vi "Win32Test.vi"() -> ()   [LabVIEW 2016]
uses:
  CAN_Info.ctl
  CAN_BaudInfo.ctl
  CAN_FrameInfo.ctl
  BusStatistics/TLIBCANBusStatistics_Ctrl.ctl
  MessageInfo.ctl
panel:
  out "tsapp_delete_cyclic_msg_can":i32
  in  "AAppChannel":i32(ring) items=["CHN1", "CHN2", "CHN3", "CHN4", "CHN5", "CHN6", "CHN7", "CHN8", "CHN9", "CHN10", "CHN11", "CHN12", "CHN13", "CHN14", "CHN15", "CHN16", "CHN17", "CHN18", "CHN19", "CHN20", "CHN21", "CHN22", "CHN23", "CHN24", "CHN25", "CHN26", "CHN27", "CHN28", "CHN29", "CHN30", "CHN31", "CHN32"]
  in  "删除周期消息":bool
  in  "周期消息":T1 {"ADLC" max=64; "AID" max=536870911}
  in  "添加周期发送消息":bool
  out "tsapp_add_cyclic_msg_can":i32
  in  "消息周期":sgl=10.0
  out "接收的数据":T2[](array[typedef])
  in  "空白按钮":bool
  in  "查询内容":u16(ring) items=["获取网络名称"=0, "获取dbc文件名"=1, "获取协议类型，0=CAN、1=J1939"=2, "获取信号表数量"=10, "获取CAN报文表数量"=11, "获取CANFD报文表数量"=12, "获取CANJ1939报文表数量"=13, "获取节点表数量"=14, "获取环境变量表数量"=15, "获取取值表数量"=16, "获取信号表中第idx信号所在的报文标识符"=20, "获取信号表中第idx信号值类型"=21, "获取信号表中第idx信号是否是Motorola"=22, "获取信号表中第idx信号所带的取值表在取值表列表中的索引"=23, "获取信号表中第idx信号Mux类型"=24, "获取信号表中第idx信号作为multiplexor的值"=25, "获取信号表中第idx信号在报文中的起始位"=26, "获取信号表中第idx信号的信号长度"=27, "获取信号表中第idx信号放大因子"=28, "获取信号表中第idx信号偏移量"=29, "获取信号表中第idx信号初始值"=30, "获取信号表中第idx信号最小值"=31, "获取信号表中第idx信号最大值"=32, "获取信号表中第idx信号名称"=33, "获取信号表中第idx信号单位"=34, "获取信号表中第idx信号注释"=35, "获取信号表中第idx信号所在的报文在报文表中的索引"=36, "获取信号表中第idx信号所在的报文的类型"=37, "获取信号表中第idx信号全部属性"=38, "获取CAN报文表中第idx报文类型"=40, "获取CAN报文表中第idx报文数据长度"=41, "获取CAN报文表中第idx报文标识符"=42, "获取CAN报文表中第idx报文周期"=43, "获取CAN报文表中第idx报文名称"=44, "获取CAN报文表中第idx报文注释"=45, "获取CAN报文表中第idx报文对应的发送节点的索引"=46, "获取CAN报文表中第idx报文拥有的信号数量"=47, "获取CAN报文表中第idx报文中第subidx信号在信号表中的索引"=48, "获取CAN报文表中第idx报文全部属性"=49, "获取CANFD报文表中第idx报文属性"=60, "获取CANFD报文表中第idx报文数据长度"=61, "获取CANFD报文表中第idx报文标识符"=62, "获取CANFD报文表中第idx报文周期"=63, "获取CANFD报文表中第idx报文名称"=64, "获取CANFD报文表中第idx报文注释"=65, "获取CANFD报文表中第idx报文对应的发送节点的索引"=66, "获取CANFD报文表中第idx报文拥有的信号数量"=67, "获取CANFD报文表中第idx报文中第subidx信号在信号表中的索引"=68, "获取CANFD报文表中第idx报文BRS"=69, "获取CANFD报文表中第idx报文全部属性"=70, "获取J1939报文表中第idx报文类型"=80, "获取J1939报文表中第idx报文数据长度"=81, "获取J1939报文表中第idx报文标识符"=82, "获取J1939报文表中第idx报文周期"=83, "获取J1939报文表中第idx报文名称"=84, "获取J1939报文表中第idx报文注释"=85, "获取J1939报文表中第idx报文对应的发送节点的索引"=86, "获取J1939报文表中第idx报文拥有的信号数量"=87, "获取J1939报文表中第idx报文中第subidx信号在信号表中的索引"=88, "获取CAN报文表中第idx报文全部属性"=89, "获取节点表中第idx节点地址"=100, "获取节点表中第idx节点名称"=101, "获取取值表中第idx取值表所包含的值数量"=140, "获取取值表中第idx取值表名称"=141, "获取取值表中第idx取值表中第subidx的值"=142, "获取取值表中第idx取值表全部属性"=143]
  in  "查询dbc":bool
  in  "清除总线统计":bool
  out "TLIBCANBusStatistics_Ctrl":T3
  in  "开启blf记录":bool
  in  "Blf文件路径":path=path "D:/LabviewWorkSpace/海卓项目资料/SFCV FCURig 文件夹/BottomLevel/TS_CANDrive/Test_blf/UserBlf.blf"
  in  "使能统计功能":bool
  out "out AId":u32
  in  "ASupportedChannelsBased0":string
  in  "路径":path
  in  "加载dbc":bool
  in  "错误输入":errorcluster caption="错误输出"
  out "错误输出":errorcluster
  out "ConnectSeccessfully":bool
  in  "初始化CAN通道":bool
  out "接收总数":i32
  in  "发送通道":i32(ring) items=["CHN1", "CHN2", "CHN3", "CHN4", "CHN5", "CHN6", "CHN7", "CHN8", "CHN9", "CHN10", "CHN11", "CHN12", "CHN13", "CHN14", "CHN15", "CHN16", "CHN17", "CHN18", "CHN19", "CHN20", "CHN21", "CHN22", "CHN23", "CHN24", "CHN25", "CHN26", "CHN27", "CHN28", "CHN29", "CHN30", "CHN31", "CHN32"]
  in  "发送数据帧信息":T1={"AID"=1234, "AIsExt"=enum."STD", "AIsRemote"=enum."Data", "ADLC"=5, "ADataArray"=[0, 0, 10, 96, 8, 8]} {"ADLC" max=64; "AID" max=536870911}
  in  "配置波特率":T4={"ABaudrateKbps"=500.0, "AListenOnly"=enum."Normal", "Int120Ohm"=enum."Enable", "EnableChannel"=enum."Enable", "AAppChannel"=0, "硬件类型"=8, "AHwChannel"=0} {"AHwChannel" items=["CHN1", "CHN2", "CHN3", "CHN4", "CHN5", "CHN6", "CHN7", "CHN8", "CHN9", "CHN10", "CHN11", "CHN12", "CHN13", "CHN14", "CHN15", "CHN16", "CHN17", "CHN18", "CHN19", "CHN20", "CHN21", "CHN22", "CHN23", "CHN24", "CHN25", "CHN26", "CHN27", "CHN28", "CHN29", "CHN30", "CHN31", "CHN32"]; "硬件类型" items=["BUS_UNKNOWN_TYPE", "TS_TCP_DEVICE", "XL_USB_DEVICE", "TS_USB_DEVICE", "PEAK_USB_DEVICE", "KVASER_USB_DEVICE", "ZLG_USB_DEVICE", "ICS_USB_DEVICE", "TS_TC1005_DEVICE"]; "AAppChannel" items=["CHN1", "CHN2", "CHN3", "CHN4", "CHN5", "CHN6", "CHN7", "CHN8", "CHN9", "CHN10", "CHN11", "CHN12", "CHN13", "CHN14", "CHN15", "CHN16", "CHN17", "CHN18", "CHN19", "CHN20", "CHN21", "CHN22", "CHN23", "CHN24", "CHN25", "CHN26", "CHN27", "CHN28", "CHN29", "CHN30", "CHN31", "CHN32"]}
  in  "CAN_CardProperties":T5={"应用程序名"="APP", "CAN使用通道数"=5, "LIN使用通道数"=0} {"LIN使用通道数" max=5; "CAN使用通道数" max=5}
  in  "停止":bool
  # "win32目前没有dbc属性获取，\n需要.net方式"
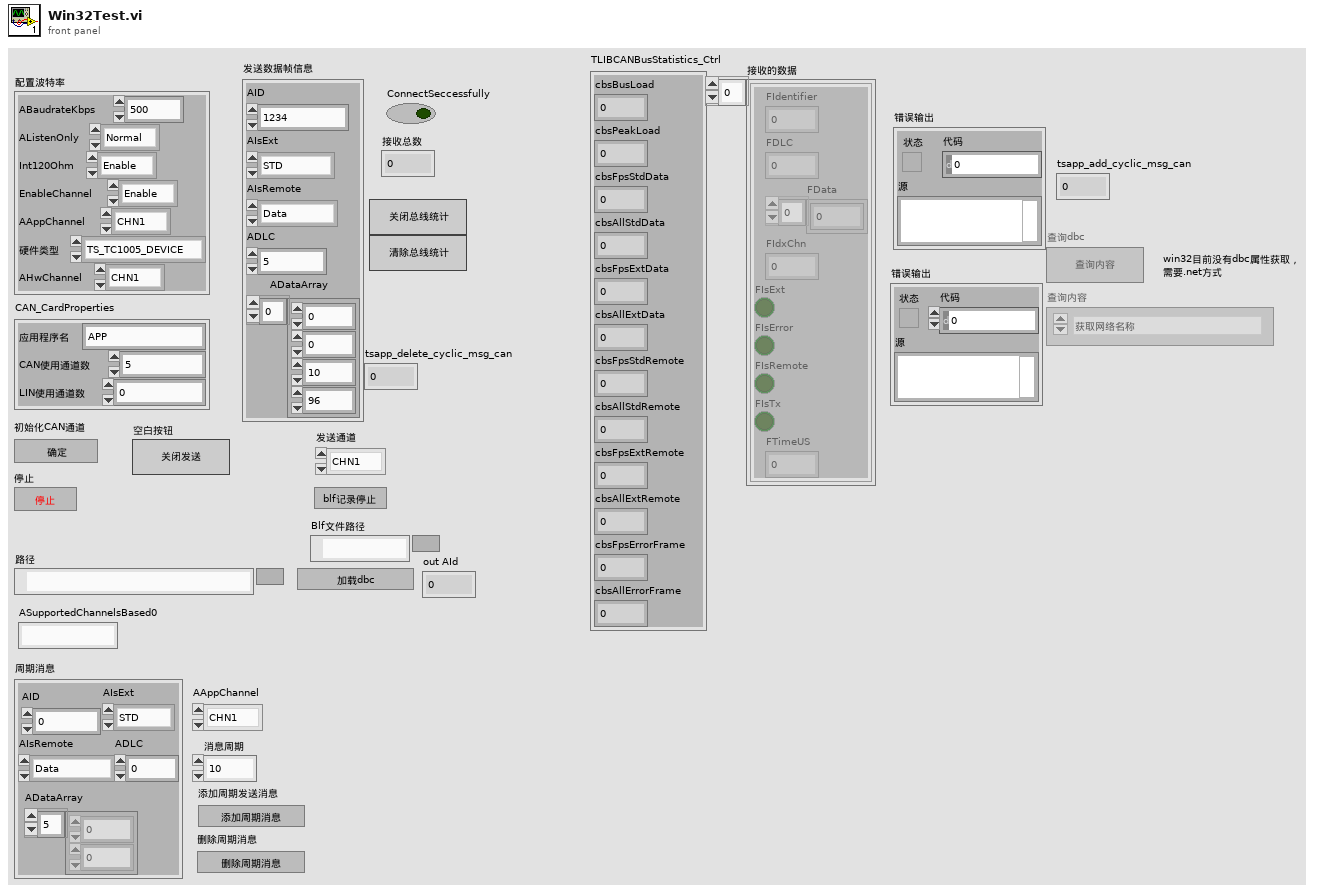
[diagram p1: front panel]
types:
  T1 = typedef "CAN_FrameInfo.ctl" = cluster{"AID":u32, "AIsExt":enum16{"STD", "EXT"}, "AIsRemote":enum16{"Data", "Remote"}, "ADLC":u8, "ADataArray":u8[]}
  T2 = typedef "MessageInfo.ctl" = cluster{"FIdentifier":i32, "FDLC":u8, "FData":u8[], "FIdxChn":u8, "FIsExt":bool, "FIsError":bool, "FIsRemote":bool, "FIsTx":bool, "FTimeUS":u64}
  T3 = typedef "TLIBCANBusStatistics_Ctrl.ctl" = cluster{"cbsBusLoad":dbl, "cbsPeakLoad":dbl, "cbsFpsStdData":dbl, "cbsAllStdData":dbl, "cbsFpsExtData":dbl, "cbsAllExtData":dbl, "cbsFpsStdRemote":dbl, "cbsAllStdRemote":dbl, "cbsFpsExtRemote":dbl, "cbsAllExtRemote":dbl, "cbsFpsErrorFrame":dbl, "cbsAllErrorFrame":dbl}
  T4 = typedef "CAN_BaudInfo.ctl" = cluster{"ABaudrateKbps":sgl, "AListenOnly":enum16{"Normal", "ListenOnly"}, "Int120Ohm":enum16{"Disable", "Enable"}, "EnableChannel":enum16{"Disable", "Enable"}, "AAppChannel":i32, "硬件类型":i32, "AHwChannel":i32}
  T5 = typedef "CAN_Info.ctl" = cluster{"应用程序名":string, "CAN使用通道数":u8, "LIN使用通道数":u8}
  T6 = enum16{"CHAN1", "CHAN2", "CHAN3", "CHAN4", "CHAN5", "CHAN6", "CHAN7", "CHAN8", "CHAN9", "CHAN10", "CHAN11", "CHAN12", "CHAN13", "CHAN14", "CHAN15", "CHAN16"}
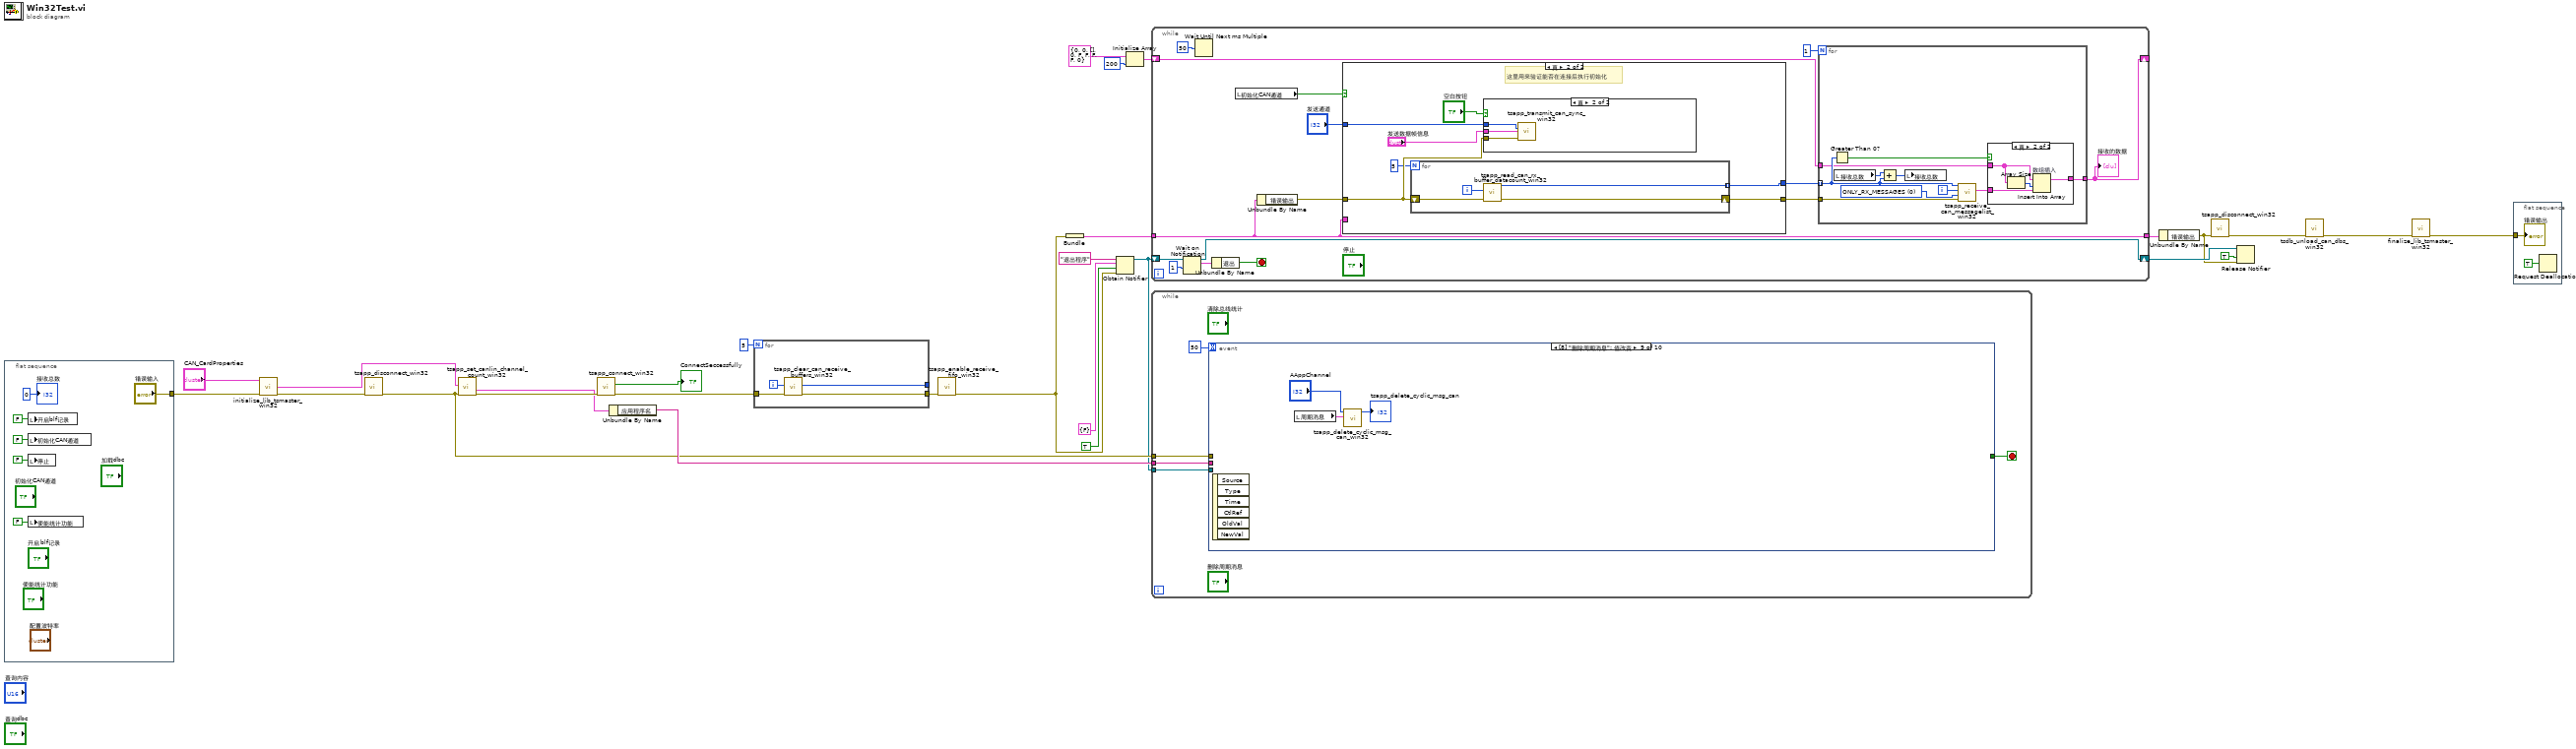
[diagram p0: block diagram]
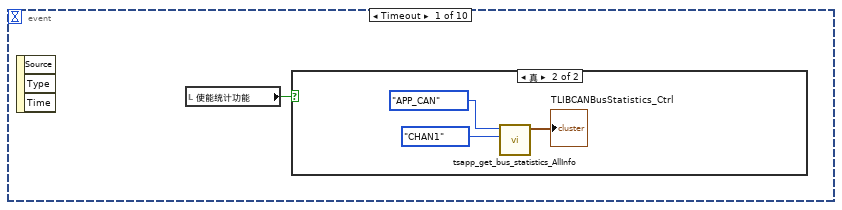
[diagram p2: hidden frame]
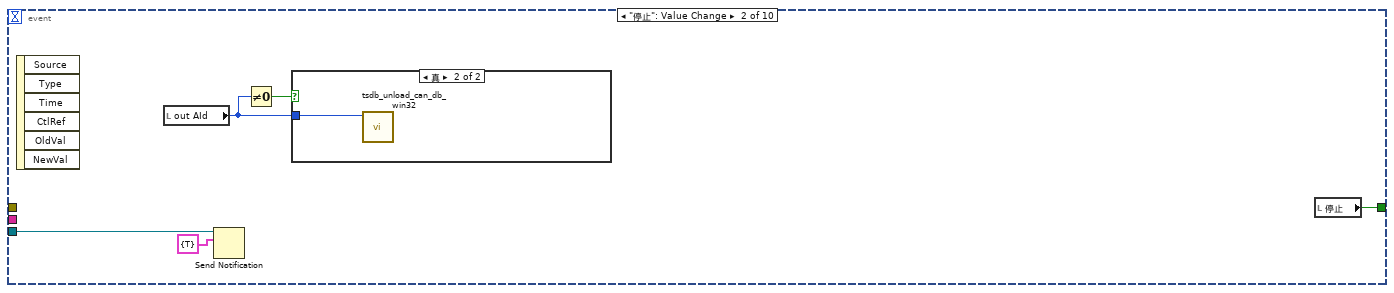
[diagram p4: hidden frame]
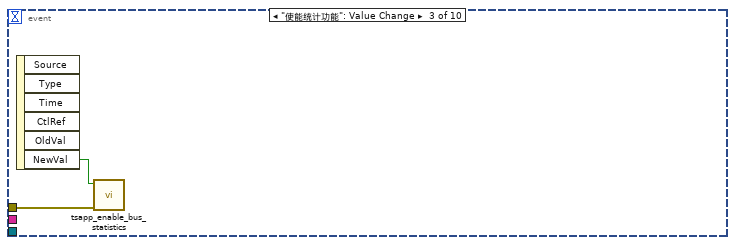
[diagram p6: hidden frame]
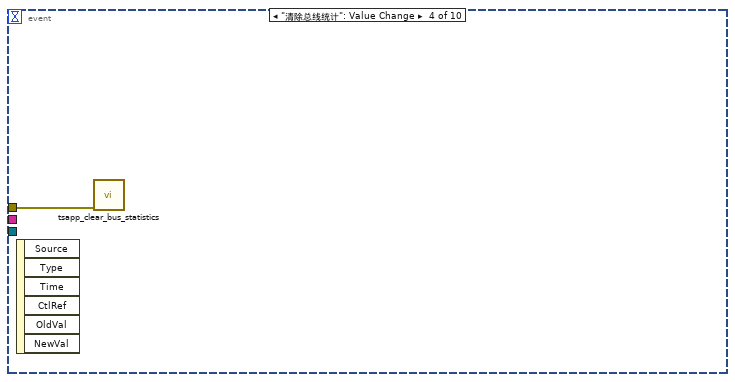
[diagram p7: hidden frame]
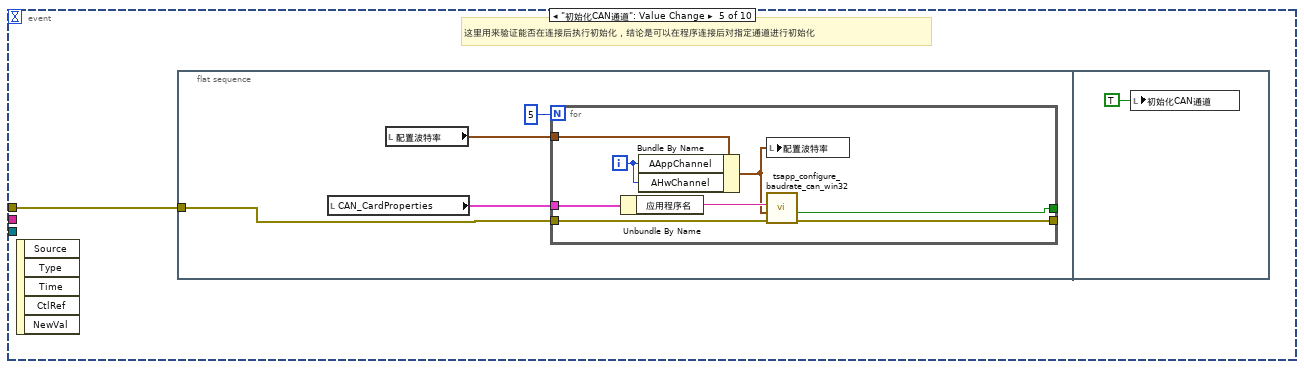
[diagram p8: hidden frame]
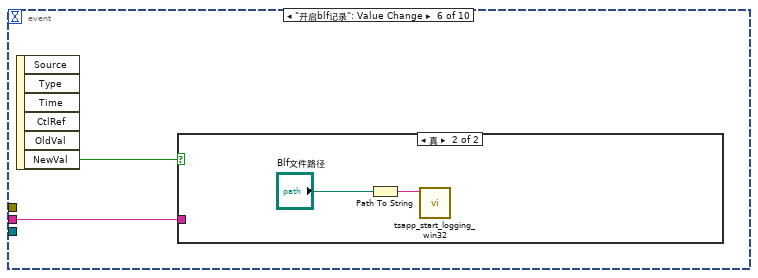
[diagram p9: hidden frame]
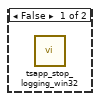
[diagram p10: hidden frame]
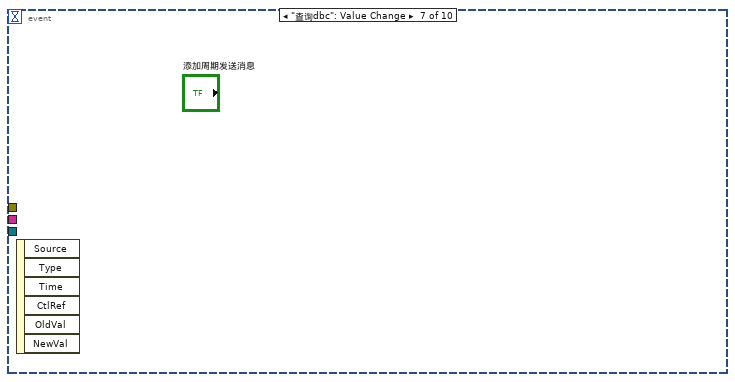
[diagram p11: hidden frame]
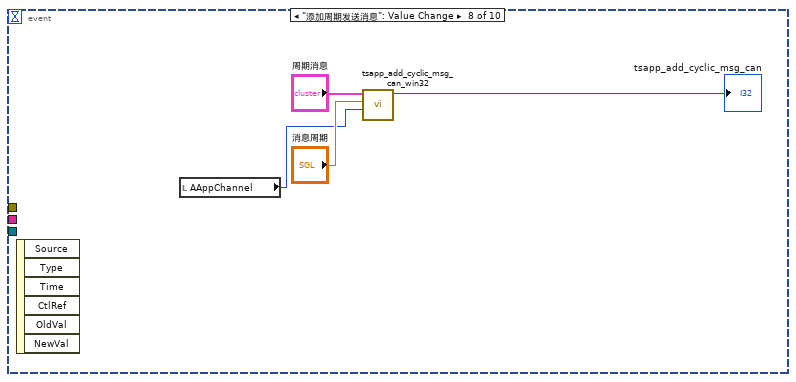
[diagram p12: hidden frame]
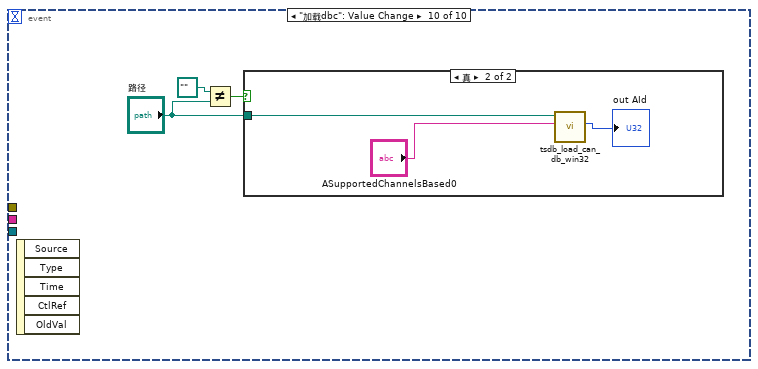
[diagram p13: hidden frame]
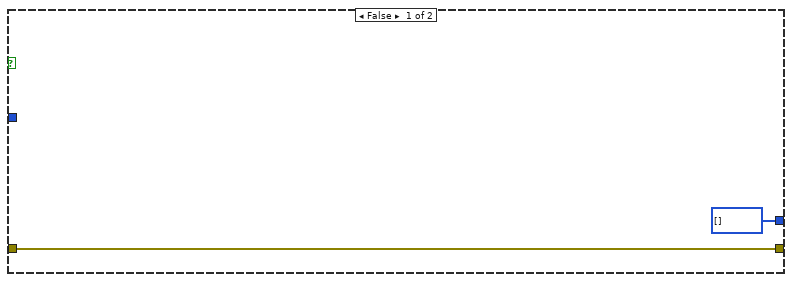
[diagram p16: hidden frame]
diagram:
  n1 = flat-sequence {
    tunnel: ["错误输入"] -> w17
    frame #0 {
      n2 = local write "开启blf记录"(FALSE ("开启blf记录")) -> ()
      n3 = local write "初始化CAN通道"(FALSE ("初始化CAN通道")) -> ()
      n4 = local write "停止"(FALSE ("停止")) -> ()
      n5 = local write "使能统计功能"(FALSE ("使能统计功能")) -> ()
      "接收总数" <- 0 ("接收总数")
    }
  }
  n6 = call "initialize_lib_tsmaster_win32.vi"("初始化CAN通道"="CAN_CardProperties", "错误输入（无错误）"=w17) -> ("InitializationInformation"=w25:T5, "错误输出"=w20:errorcluster)  [unwired: 10 in, 2 out]
  n7 = call "tsapp_disconnect_win32.vi"("错误输入（无错误）"=w20) -> ("错误输出"=w12:errorcluster)  [unwired: 8 in, 2 out]
  n8 = call "tsapp_set_canlin_channel_count_win32.vi"("错误输入（无错误）"=w12, "InitializationInformation"=w25) -> ("错误输出"=w19:errorcluster, "InitializationInformation_Out"=w16:T5)  [unwired: 7 in, 1 out]
  n9 = call "tsapp_connect_win32.vi"("错误输入（无错误）"=w19) -> ("错误输出"=w24:errorcluster, "ConnectSeccessfully"=→"ConnectSeccessfully":bool)  [unwired: 8 in, 1 out]
  n10 = Unbundle By Name(w16) -> ("应用程序名"=w15:string)
  n11 = for {
    N: 5 -> [_]
    tunnel: [w36] -> _
    tunnel: w24 -> [w38]
    tunnel: [w37] -> w23
    i -> [w35]
    n12 = call "tsapp_clear_can_receive_buffers_win32.vi"("错误输入（无错误）"=w38, "AAppChannel"=w35) -> ("错误输出"=w37:errorcluster, "tsapp_clear_can_receive_buffers"=w36:i32)  [unwired: 8 in]
  }
  n13 = call "tsapp_enable_receive_fifo_win32.vi"("错误输入（无错误）"=w23) -> ("错误输出"=w8:errorcluster)  [unwired: 10 in]
  n14 = Bundle("错误输出"=w8) -> (w28:cluster{"错误输出":errorcluster})  [unwired: 1 in]
  n15 = Obtain Notifier(name (unnamed)="退出程序" ("名称（未命名）"), notification data type=cluster{"退出":bool} {"退出"=FALSE} ("退出程序"), create if not found? (T)=TRUE ("如未找到则创建？(T)"), error in (no error)=w8) -> (notifier out=w4:refnum<notifier>)  [unwired: 2 out]
  n16 = Initialize Array(T2 {"FIdentifier"=0, "FDLC"=0, "FData"=[], "FIdxChn"=0, "FIsExt"=FALSE, "FIsError"=FALSE, "FIsRemote"=FALSE, "FIsTx"=FALSE, "FTimeUS"=0} ("Receive message"), 200 ("维数大小")) -> (w1:T2[])
  n17 = while {
    tunnel: w28 -> [w53]
    tunnel: [w53] -> w27
    shift-right: [w39] -> _
    shift-left: w1 -> [w51]
    shift-right: [w42] -> w7
    shift-left: w4 -> [w44]
    stop <- w40 stop-if-true
    n18 = Wait on Notification(notifier=w44, timeout in ms (-1)=1 ("超时毫秒(-1)")) -> (notifier out=w42:refnum<notifier>, notification=w41:cluster{"退出":bool})  [unwired: 2 in, 2 out]
    n19 = Wait Until Next ms Multiple(millisecond multiple=u32 50 ("毫秒倍数")) -> ()  [unwired: 1 out]
    n20 = Unbundle By Name(w41) -> ("退出"=w40:bool)
    n21 = local read "初始化CAN通道"() -> (w49:bool)
    n22 = Unbundle By Name(w53) -> ("错误输出"=w48:errorcluster)
    n23 = case shown="真" w49 {
      tunnel: w53 -> [_ _]
      tunnel: [w70 w77] -> w52
      tunnel: [i32[] [] w76] -> w50
      tunnel: "发送通道" -> [_ w74]
      tunnel: w48 -> [w70 w75]
      frame False {
      }
      frame True {
        # "这里用来验证能否在连接后执行初始化"
        n24 = for {
          N: 5 -> [_]
          tunnel: [w83] -> w76 mode=indexing
          shift-right: [w84] -> w77
          shift-left: w75 -> [w82]
          i -> [w81]
          n25 = call "tsapp_read_can_rx_buffer_datacount_win32.vi"("错误输入（无错误）"=w82, "AAppChannel"=w81) -> ("错误输出"=w84:errorcluster, "tsapp_read_can_buffer_datacount"=w83:i32)  [unwired: 7 in, 1 out]
        }
        n26 = case shown="真" "空白按钮" {
          tunnel: w75 -> [_ w80]
          tunnel: w74 -> [_ w79]
          tunnel: "发送数据帧信息" -> [_ w78]
          frame False {
          }
          frame True {
            n27 = call "tsapp_transmit_can_sync_win32.vi"("AAppChannel"=w79, "数据帧信息"=w78, "错误输入（无错误）"=w80) -> ()  [unwired: 10 in, 3 out]
          }
        }
      }
    }
    n28 = for {
      N: 1 -> [_]
      tunnel: w52 -> [w63]
      tunnel: w50 -> [w61] mode=indexing
      tunnel: w51 -> [w55]
      tunnel: [w54] -> w39
      i -> [w62]
      w57 = u8 0 items=["ONLY_RX_MESSAGES", "TX_RX_MESSAGES"] ("AOnlyRx")
      n29 = Greater Than 0?(x=w61) -> (x > 0?=w56:bool)
      n30 = local read "接收总数"() -> (w60:i32)
      n31 = Add(x=w60, y=w61) -> (x+y=w59:i32)
      n32 = local write "接收总数"(w59) -> ()
      n33 = call "tsapp_receive_can_messagelist_win32.vi"("错误输入（无错误）"=w63, "AOnlyRx"=w57, "AAppChannel输入"=w62, "ACANBufferSize"=w61) -> ("tsapp_receive_can_messageList"=w58:T2[])  [unwired: 5 in, 2 out]
      n34 = case shown="真" w56 {
        tunnel: w58 -> [_ w68]
        tunnel: w55 -> [w64 w67]
        tunnel: [w64 w65] -> w54
        frame False {
        }
        frame True {
          n35 = Array Size(array=w67) -> (size(s)=w66:i32)
          n36 = Insert Into Array "数组插入"(array=w67, index=w66, new element=w68) -> (w65:T2[])
        }
      }
    }
    "接收的数据" <- w39
  }
  n37 = while {
    tunnel: w12 -> [w89]
    tunnel: w15 -> [w86]
    tunnel: w4 -> [w85]
    stop <- w87 stop-if-true
    n38 = event shown="[8] \"删除周期消息\": 值改变" {
      selector: _ -> [_ _ _ _ _ _ _ _ _ _]
      dyn-events: _ -> [_ _ _ _ _ _ _ _ _ _]
      timeout: 50 -> [_ _ _ _ _ _ _ _ _ _]
      tunnel: w89 -> [_ _ w100 w102 w103 _ _ _ _ _]
      tunnel: [_ w98 _ _ _ _ _ _ _ _] -> w87
      tunnel: w86 -> [_ _ _ _ _ w117 _ _ _ _]
      tunnel: w85 -> [_ w95 _ _ _ _ _ _ _ _]
      event Timeout {
        n39 = event-data() -> ()  [unwired: 1 in, 3 out]
        n40 = local read "使能统计功能"() -> (w90:bool)
        n41 = case shown="真" w90 {
          frame False {
          }
          frame True {
            n42 = call "tsapp_get_bus_statistics_AllInfo.vi"("AIdxChn"=T6."CHAN1", "ABusType"=enum16{"APP_CAN", "APP_LIN"}."APP_CAN") -> ("TLIBCANBusStatistics_Ctrl"=→"TLIBCANBusStatistics_Ctrl":T3)  [unwired: 8 in, 1 out]
          }
        }
      }
      event "停止": Value Change {
        n43 = event-data() -> ()  [unwired: 1 in, 6 out]
        n44 = local read "out AId"() -> (w97:u32)
        n45 = Send Notification(notification=cluster{"退出":bool} {"退出"=TRUE} ("通知"), notifier=w95) -> ()  [unwired: 1 in, 2 out]
        n46 = Not Equal To 0?(x=w97) -> (x != 0?=w96:bool)
        n47 = case shown="真" w96 {
          tunnel: w97 -> [_ w99]
          frame False {
          }
          frame True {
            n48 = call "tsdb_unload_can_db_win32.vi"("out AId"=w99) -> ()  [unwired: 9 in, 2 out]
          }
        }
        n49 = local read "停止"() -> (w98:bool)
      }
      event "使能统计功能": Value Change {
        n50 = event-data() -> ("NewVal"=w101:bool)  [unwired: 1 in, 5 out]
        n51 = call "tsapp_enable_bus_statistics.vi"("错误输入（无错误）"=w100, "Enable"=w101) -> ()  [unwired: 8 in, 2 out]
      }
      event "清除总线统计": Value Change {
        n52 = event-data() -> ()  [unwired: 1 in, 6 out]
        n53 = call "tsapp_clear_bus_statistics.vi"("错误输入（无错误）"=w102) -> ()  [unwired: 9 in, 2 out]
      }
      event "初始化CAN通道": Value Change {
        # "这里用来验证能否在连接后执行初始化，结论是可以在程序连接后对指定通道进行初始化"
        n54 = event-data() -> ()  [unwired: 1 in, 5 out]
        n55 = flat-sequence {
          tunnel: w103 -> [w105]
          frame #0 {
            n56 = local read "CAN_CardProperties"() -> (w106:T5)
            n57 = local read "配置波特率"() -> (w107:T4)
            n58 = for {
              N: 5 -> [_]
              tunnel: w106 -> [w112]
              tunnel: [w114] -> _
              tunnel: w105 -> [w115]
              tunnel: [w113] -> _
              tunnel: w107 -> [w110]
              i -> [w109]
              n59 = Unbundle By Name(w112) -> ("应用程序名"=w111:string)
              n60 = Bundle By Name(cluster=w110, "AAppChannel"=w109, "AHwChannel"=w109) -> (w108:T4)
              n61 = local write "配置波特率"(w108) -> ()
              n62 = call "tsapp_configure_baudrate_can_win32.vi"("AppName"=w111, "配置波特率"=w108, "错误输入（无错误）"=w115) -> ("InitSts"=w114:bool, "错误输出"=w113:errorcluster)  [unwired: 6 in]
            }
          }
          frame #1 {
            n63 = local write "初始化CAN通道"(TRUE ("初始化CAN通道")) -> ()
          }
        }
      }
      event "开启blf记录": Value Change {
        n64 = event-data() -> ("NewVal"=w118:bool)  [unwired: 1 in, 5 out]
        n65 = case shown="真" w118 {
          tunnel: w117 -> [_ _]
          frame False {
            n66 = call "tsapp_stop_logging_win32.vi"() -> ()  [unwired: 10 in, 2 out]
          }
          frame True {
            n67 = Path To String(path="Blf文件路径") -> (string=w119:string)
            n68 = call "tsapp_start_logging_win32.vi"("AFileName"=w119) -> ()  [unwired: 9 in, 2 out]
          }
        }
      }
      event "查询dbc": Value Change {
        n69 = event-data() -> ()  [unwired: 1 in, 6 out]
      }
      event "添加周期发送消息": Value Change {
        n70 = event-data() -> ()  [unwired: 1 in, 6 out]
        n71 = local read "AAppChannel"() -> (w121:i32)
        n72 = call "tsapp_add_cyclic_msg_can_win32.vi"("AAppChannel"=w121, "APeriodMS"="消息周期", "数据帧信息"="周期消息") -> ("tsapp_add_cyclic_msg_can"=→"tsapp_add_cyclic_msg_can":i32)  [unwired: 7 in, 1 out]
      }
      event "删除周期消息": Value Change {
        n73 = event-data() -> ()  [unwired: 1 in, 6 out]
        n74 = local read "周期消息"() -> (w125:T1)
        n75 = call "tsapp_delete_cyclic_msg_can_win32.vi"("数据帧信息"=w125, "AAppChannel"="AAppChannel") -> ("tsapp_delete_cyclic_msg_can"=→"tsapp_delete_cyclic_msg_can":i32)  [unwired: 8 in, 1 out]
      }
      event "加载dbc": Value Change {
        n76 = event-data() -> ()  [unwired: 1 in, 5 out]
        n77 = Not Equal?(x=path "", y="路径") -> (x != y?=w129:bool)
        n78 = case shown="真" w129 {
          tunnel: "路径" -> [_ w132]
          frame False {
          }
          frame True {
            n79 = call "tsdb_load_can_db_win32.vi"("ASupportedChannelsBased0"="ASupportedChannelsBased0", "路径"=w132) -> ("out AId"=→"out AId":u32)  [unwired: 7 in, 2 out]
          }
        }
      }
    }
  }
  n80 = Unbundle By Name(w27) -> ("错误输出"=w5:errorcluster)
  n81 = call "tsapp_disconnect_win32.vi"("错误输入（无错误）"=w5) -> ("错误输出"=w14:errorcluster)  [unwired: 8 in, 2 out]
  n82 = Release Notifier(notifier=w7, force destroy? (F)=TRUE ("强制销毁？(F)"), error in (no error)=w5) -> ()  [unwired: 3 out]
  n83 = call "tsdb_unload_can_dbs_win32.vi"("错误输入（无错误）"=w14) -> ("错误输出"=w13:errorcluster)  [unwired: 9 in, 1 out]
  n84 = call "finalize_lib_tsmaster_win32.vi"("错误输入（无错误）"=w13) -> ("错误输出"=w18:errorcluster)  [unwired: 10 in]
  n85 = flat-sequence {
    tunnel: w18 -> [w135]
    frame #0 {
      n86 = Request Deallocation(TRUE ("标志")) -> ()
      "错误输出" <- w135
    }
  }
